vi "Actor Core.vi"(8 "Error in":errorcluster, 11 "Nested in":refnum<class "Protocol Verification Test.lvclass">) -> (0 "error out":errorcluster, 3 "Actor out":refnum<class "Actor.lvclass">)   [LabVIEW 2017, in "Protocol Verification Test.lvlib" / "Protocol Verification Test.lvclass"]
doc: "(<B>Filename</B>: Actor Framework.lvlib:Actor.lvclass:Actor Core.vi)\n\nReceives messages to the actor, reacts to them, and initiates any error handling that may shut the actor down.\n\nDescendant classes may override this VI to append parallel tasks for the actor to complete while it handles messages. Overrides use the Call Parent Method node."
uses:
  Protocol Verification Test.lvclass
  C:/Program Files (x86)/National Instruments/LabVIEW 2017/vi.lib/ActorFramework/Actor/Actor.lvclass
  <vilib>/ActorFramework/Actor/Actor.lvclass
  Proto Test Helper Loop States.ctl
  <vilib>/ActorFramework/Message Enqueuer/Message Enqueuer.lvclass
  TLV Data.ctl
  Protocol Verification Configuration.ctl
  Protocol Verification Test.lvclass/Protocol Verification Test.ctl
  <vilib>/ActorFramework/Actor/Actor.lvclass/Actor.ctl
  <vilib>/ActorFramework/Message Enqueuer/Message Enqueuer.lvclass/Message Enqueuer.ctl
  Test/Test Messages/Update Test Progress Msg/Update Test Progress Msg.lvclass/Update Test Progress Msg.ctl
  Protocol Verification Test Messages/TLV Frame Msg/TLV Frame Msg.lvclass/TLV Frame Msg.ctl
  Protocol Verification Test Messages/Write Proto Test Configuration Msg/Write Proto Test Configuration Msg.lvclass/Write Proto Test Configuration Msg.ctl
  <vilib>/ActorFramework/Message Enqueuer/Init from Existing Queue.vi
  <vilib>/ActorFramework/Message Enqueuer/Enqueue.vi
  Test/Test Messages/Update Test Progress Msg/Update Test Progress Msg.lvclass
  C:/Program Files (x86)/National Instruments/LabVIEW 2017/vi.lib/ActorFramework/Message/Message.lvclass
  Protocol Verification Test Messages/TLV Frame Msg/TLV Frame Msg.lvclass
  Protocol Verification Test Messages/Write Proto Test Configuration Msg/Write Proto Test Configuration Msg.lvclass
  <vilib>/ActorFramework/Message Priority Queue/Priority Enqueue.vi
  Test/Test/Test.lvclass
  Protocol Verification Test.lvlib
panel:
  out "Protocol Test":i32[](listbox)
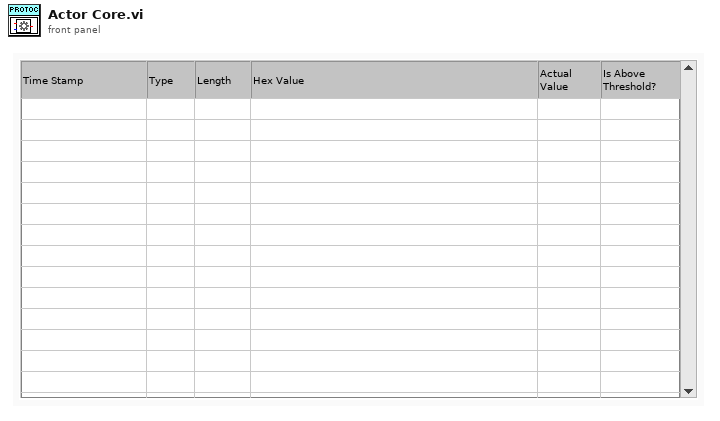
[diagram p1: front panel]
types:
  T1 = typedef "Protocol Verification Test.lvlib/TLV Data.ctl" = cluster{"Type":u8, "Length":u8, "Value":u8[]}
  T2 = typedef "Protocol Verification Test.lvlib/Protocol Verification Configuration.ctl" = cluster{"Type To Filter":i32, "Threshold":dbl, "Binary File Path":path}
  T3 = cluster{"raw bytes":u8[], "Self Enqueuer":refnum<class "Message Enqueuer.lvclass">, "TLV Data":T1[], "Test Name":string, "Protocol Verification Data":T2}
  T4 = typedef "Protocol Verification Test.lvlib/Protocol Verification Test.lvclass/Proto Test Helper Loop States.ctl" = enum16{"Poll", "Init", "Read Test Case", "Update Test Case to Actor", "Read Input File", "Parse Data", "Stream Data to Actor", "Mark End Of Stream", "Update Result", "Update Report", "Error", "Exit"}
  T5 = cluster{"Type To Filter":i32, "Threshold":dbl, "Binary File Path":string}
  T6 = typedef "Paths.ctl" = cluster{"Data Directory":path, "Test Config Dir":path, "Error Logs":path, "Event Logs":path, "Settings.Json":path, "Reports Directory":path}
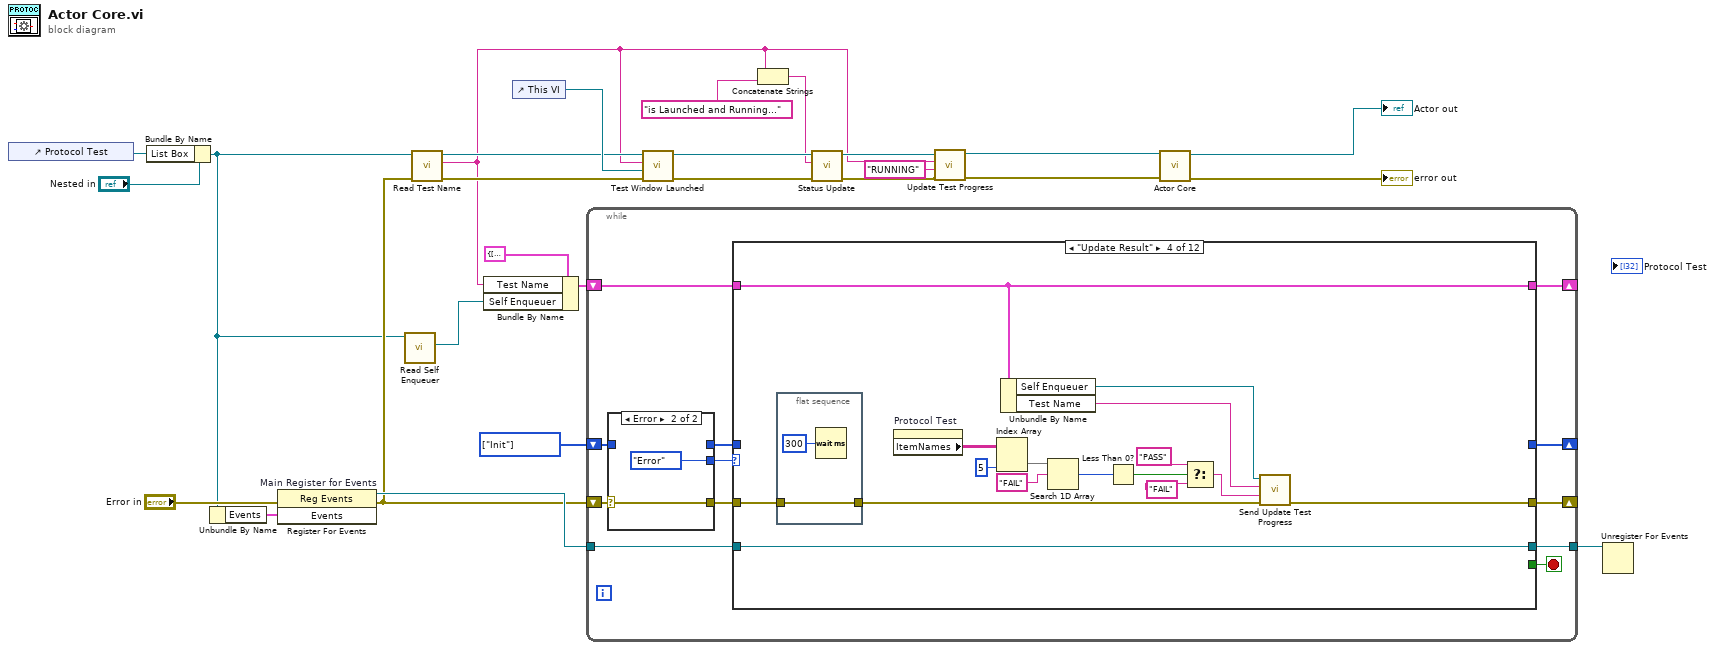
[diagram p0: block diagram]
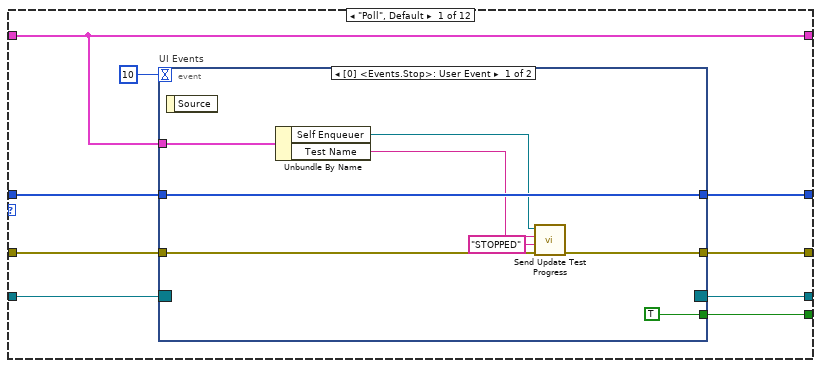
[diagram p2: hidden frame]
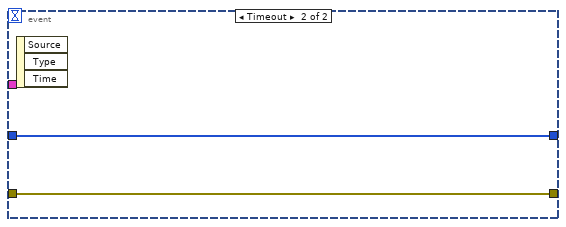
[diagram p3: hidden frame]
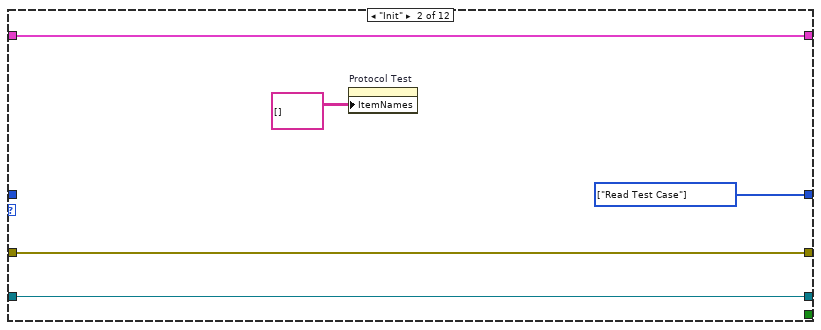
[diagram p4: hidden frame]
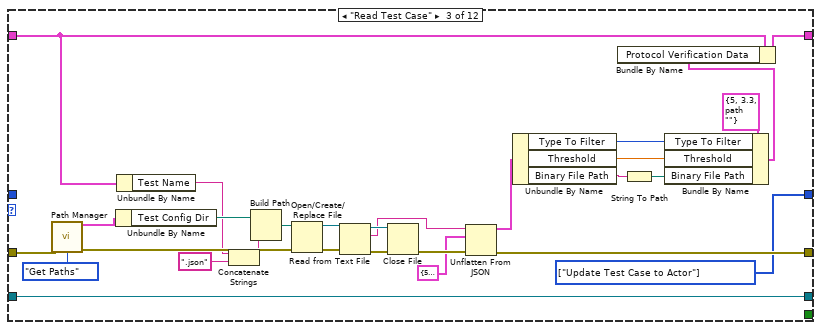
[diagram p5: hidden frame]
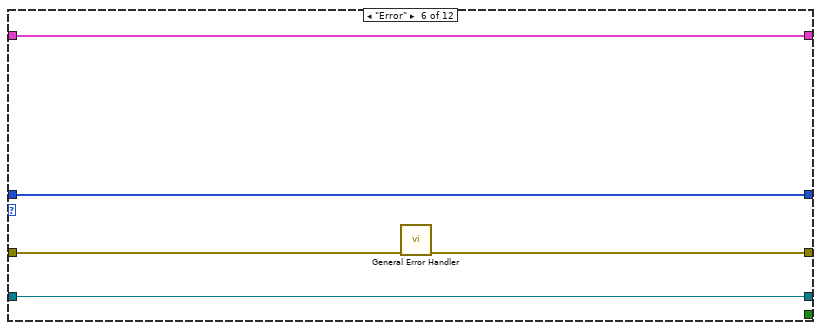
[diagram p7: hidden frame]
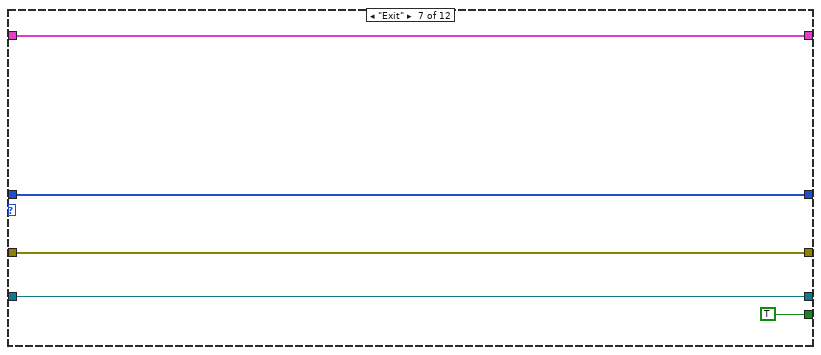
[diagram p8: hidden frame]
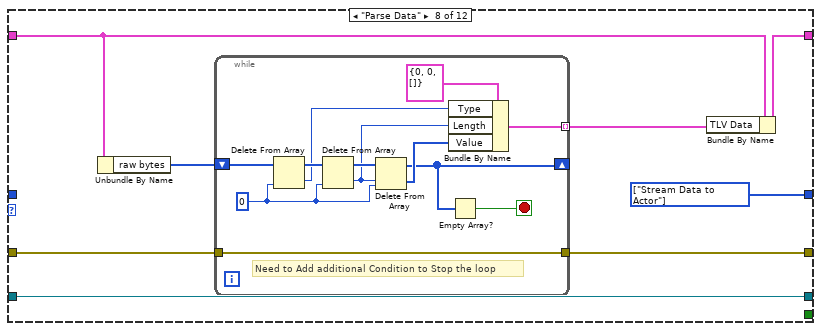
[diagram p9: hidden frame]
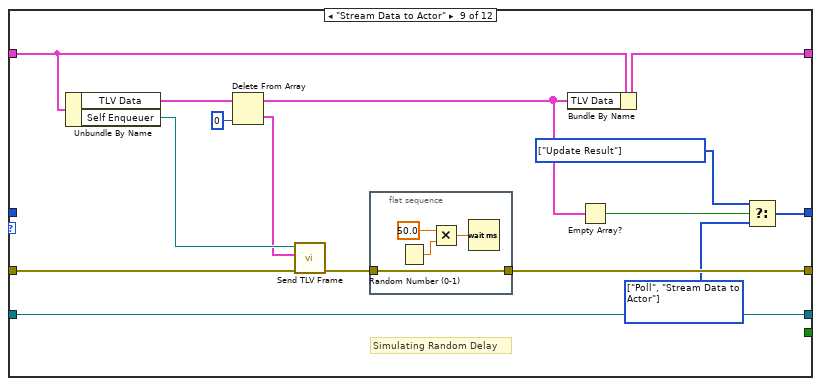
[diagram p10: hidden frame]
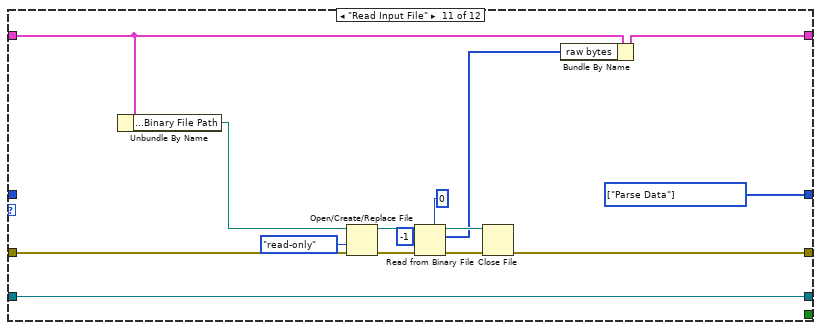
[diagram p12: hidden frame]
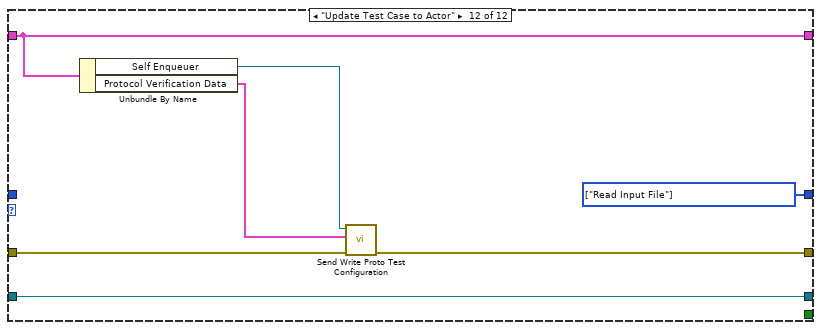
[diagram p13: hidden frame]
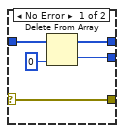
[diagram p14: hidden frame]
diagram:
  w19 = T4[] [enum."Init"] items=["Poll", "Init", "Read Test Case", "Update Test Case to Actor", "Read Input File", "Parse Data", "Stream Data to Actor", "Mark End Of Stream", "Update Result", "Update Report", "Error", "Exit"]
  n1 = control-ref of="Protocol Test"() -> (w18:refnum<vi>)
  n2 = Bundle By Name(cluster="Nested in", "List Box"=w18) -> (w5:refnum<class "Protocol Verification Test.lvclass">)
  n3 = Unbundle By Name(w5) -> ("Events"=w24:cluster{"Stop":refnum<user-event>})
  n4 = register-events "Main Register for Events"(error in="Error in", w24) -> (reference out=w25:refnum<event-registration>, error out=w7:errorcluster)  [unwired: 1 in]
  n5 = call <vilib>:"Read Self Enqueuer.vi"("Actor"=w5) -> ("Self Enqueuer"=w11:refnum<class "Message Enqueuer.lvclass">)  [unwired: 10 in]
  n6 = call-dynamic "Read Test Name.vi"("error in (no error)"=w7, "Test in"=w5) -> ("error out"=w6:errorcluster, "Test Name"=w1:string, "Test out"=w4:refnum<class "Protocol Verification Test.lvclass">)  [unwired: 7 in]
  n7 = Bundle By Name(cluster=T3 {"raw bytes"=[], "Self Enqueuer"=refnum, "TLV Data"=[], "Test Name"="", "Protocol Verification Data"={"Type To Filter"=5, "Threshold"=3.3, "Binary File Path"=path ""}}, "Test Name"=w1, "Self Enqueuer"=w11) -> (w12:T3)
  n8 = control-ref of="This VI"() -> (w21:refnum<vi>)
  n9 = while {
    tunnel: w25 -> [w39]
    tunnel: [w37] -> w23
    shift-right: [w33] -> _
    shift-left: w7 -> [w36]
    shift-right: [w32] -> _
    shift-left: w19 -> [w34]
    shift-right: [w30] -> _
    shift-left: w12 -> [w31]
    stop <- w38 stop-if-true
    n10 = case shown="Error" w36 {
      selector: w36 -> [w191 w193]
      tunnel: [w191 w193] -> w35
      tunnel: w34 -> [w190 _]
      tunnel: [w189 _] -> w28
      tunnel: [w188 Proto_Test_Helper_Loop_States."Error"] -> w29
      frame No Error {
        n11 = Delete From Array(array=w190, index=0) -> (deleted portion=w188:T4, array with subset deleted=w189:T4[])  [unwired: 1 in]
      }
      frame Error {
      }
    }
    n12 = case shown="\"Update Result\"" w29 {
      tunnel: w39 -> [w48 w63 w91 w107 w112 w117 w121 w130 w157 w164 w179 w186]
      tunnel: [w47 _ _ _ _ _ TRUE _ _ _ _ _] -> w38
      tunnel: [w46 w63 w91 w107 w112 w117 w121 w130 w157 w164 w179 w186] -> w37
      tunnel: w35 -> [w45 w62 w74 w93 _ w114 w120 w128 w150 _ w171 w185]
      tunnel: [w43 w62 w75 w106 _ w113 w120 w126 w147 _ w172 w181] -> w33
      tunnel: [w41 w60 w64 _ w110 w115 w118 w123 w144 w163 w168 w180] -> w32
      tunnel: w31 -> [w40 w59 w77 w105 w111 w116 w119 w129 w156 w162 w167 w184]
      tunnel: [w40 w59 w66 w105 w111 w116 w119 w125 w155 w162 w170 w184] -> w30
      tunnel: w28 -> [w42 _ _ _ w110 w115 w118 _ _ w163 _ _]
      frame "Poll", Default {
        n13 = event "UI Events" shown="[0] <Events.Stop>: User Event" {
          selector: w48 -> [_ _]
          dyn-events: [_ _] -> w46
          timeout: 10 -> [_ _]
          tunnel: [TRUE _] -> w47
          tunnel: w45 -> [w52 w58]
          tunnel: [w51 w58] -> w43
          tunnel: w42 -> [w55 w57]
          tunnel: [w55 w57] -> w41
          tunnel: w40 -> [w50 _]
          event User Event {
            n14 = event-data() -> ()  [unwired: 1 in, 1 out]
            n15 = Unbundle By Name(w50) -> ("Self Enqueuer"=w54:refnum<class "Message Enqueuer.lvclass">, "Test Name"=w53:string)
            n16 = call "Send Update Test Progress.vi"("error in (no error)"=w52, "State"="STOPPED", "Test Name"=w53, "Message Enqueuer"=w54) -> ("error out"=w51:errorcluster)  [unwired: 6 in, 1 out]
          }
          event Timeout {
            n17 = event-data() -> ()  [unwired: 1 in, 3 out]
          }
        }
      }
      frame "Init" {
        w60 = T4[] [enum."Read Test Case"] items=["Poll", "Init", "Read Test Case", "Update Test Case to Actor", "Read Input File", "Parse Data", "Stream Data to Actor", "Mark End Of Stream", "Update Result", "Update Report", "Error", "Exit"]
        n18 = property on="Protocol Test" class="MCListbox (strict)"("ItemNames"=string[][] [] ("Item Names")) -> ()  [unwired: 2 in, 2 out]
      }
      frame "Read Test Case" {
        w64 = T4[] [enum."Update Test Case to Actor"] items=["Poll", "Init", "Read Test Case", "Update Test Case to Actor", "Read Input File", "Parse Data", "Stream Data to Actor", "Mark End Of Stream", "Update Result", "Update Report", "Error", "Exit"] ("f")
        n19 = call "Path Manager.vi"("Error in (no error)"=w74, "Options"=enum16{"Get Paths", "Init Paths"}."Get Paths") -> ("Cluster"=w82:T6, "Error out"=w84:errorcluster)  [unwired: 12 in]
        n20 = Unbundle By Name(w82) -> ("Test Config Dir"=w81:path)
        n21 = Unbundle By Name(w77) -> ("Test Name"=w76:string)
        n22 = Concatenate Strings(w76, ".json" ("string")) -> (w80:string)
        n23 = Build Path(base path=w81, name or relative path=w80) -> (appended path=w78:path)
        n24 = Open/Create/Replace File(file path (use dialog)=w78, error in=w84) -> (refnum out=w90:refnum<file>, error out=w87:errorcluster)  [unwired: 4 in, 1 out]
        n25 = Read from Text File(file (use dialog)=w90, error in=w87) -> (refnum out=w88:refnum<file>, text=w85:string, error out=w89:errorcluster)  [unwired: 2 in, 1 out]
        n26 = Close File(refnum=w88, error in=w89) -> (error out=w86:errorcluster)  [unwired: 1 out]
        n27 = Unflatten From JSON(JSON string=w85, type and defaults=T5 {"Type To Filter"=5, "Threshold"=3.3, "Binary File Path"=""} ("Cluster"), error in (no error)=w86) -> (value=w71:T5, error out=w75:errorcluster)  [unwired: 4 in]
        n28 = Unbundle By Name(w71) -> ("Type To Filter"=w70:i32, "Threshold"=w69:dbl, "Binary File Path"=w68:string)
        n29 = String To Path(string=w68) -> (path=w67:path)
        n30 = Bundle By Name(cluster=T2 {"Type To Filter"=5, "Threshold"=3.3, "Binary File Path"=path ""} ("Cluster"), "Type To Filter"=w70, "Threshold"=w69, "Binary File Path"=w67) -> (w65:T2)
        n31 = Bundle By Name(cluster=w77, "Protocol Verification Data"=w65) -> (w66:T3)
      }
      frame "Update Result" {
        n32 = flat-sequence {
          tunnel: w93 -> [w109]
          tunnel: [w109] -> w92
          frame #0 {
            n33 = Wait (ms)(milliseconds to wait=u32 300) -> ()  [unwired: 1 out]
          }
        }
        n34 = property on="Protocol Test" class="MCListbox (strict)"() -> ("ItemNames"=w102:string[][])  [unwired: 2 in, 2 out]
        n35 = Index Array(array=w102, index (col)=5 ("disabled index (col)")) -> (element=w100:string[])  [unwired: 1 in]
        n36 = Unbundle By Name(w105) -> ("Self Enqueuer"=w104:refnum<class "Message Enqueuer.lvclass">, "Test Name"=w103:string)
        n37 = Search 1D Array(1D array=w100, element="FAIL") -> (index of element=w98:i32)  [unwired: 1 in]
        n38 = Less Than 0?(x=w98) -> (x < 0?=w97:bool)
        n39 = Select(t="PASS" ("State"), s=w97, f="FAIL" ("State")) -> (s? t:f=w94:string)
        n40 = call "Send Update Test Progress.vi"("error in (no error)"=w92, "State"=w94, "Test Name"=w103, "Message Enqueuer"=w104) -> ("error out"=w106:errorcluster)  [unwired: 6 in, 1 out]
      }
      frame "Update Report" {
      }
      frame "Error" {
        n41 = call <vilib>:"General Error Handler.vi"("error in (no error)"=w114) -> ("error out"=w113:errorcluster)  [unwired: 10 in, 4 out]
      }
      frame "Exit" {
      }
      frame "Parse Data" {
        w123 = T4[] [enum."Stream Data to Actor"] items=["Poll", "Init", "Read Test Case", "Update Test Case to Actor", "Read Input File", "Parse Data", "Stream Data to Actor", "Mark End Of Stream", "Update Result", "Update Report", "Error", "Exit"] ("f")
        n42 = Unbundle By Name(w129) -> ("raw bytes"=w127:u8[])
        n43 = while {
          tunnel: w128 -> [w134]
          shift-right: [w131] -> _
          shift-left: w127 -> [w141]
          tunnel: [w134] -> w126
          tunnel: [w133] -> w124 mode=indexing
          stop <- w138 stop-if-true
          w142 = 0 ("index")
          # "Need to Add additional Condition to Stop the loop"
          n44 = Delete From Array(array=w141, index=w142) -> (deleted portion=w136:u8, array with subset deleted=w140:u8[])  [unwired: 1 in]
          n45 = Delete From Array(array=w140, index=w142) -> (deleted portion=w135:u8, array with subset deleted=w139:u8[])  [unwired: 1 in]
          n46 = Delete From Array(array=w139, length=w135, index=w142) -> (deleted portion=w132:u8[], array with subset deleted=w131:u8[])
          n47 = Bundle By Name(cluster=T1 {"Type"=0, "Length"=0, "Value"=[]} ("Cluster"), "Type"=w136, "Length"=w135, "Value"=w132) -> (w133:T1)
          n48 = Empty Array?(array=w131) -> (empty?=w138:bool)
        }
        n49 = Bundle By Name(cluster=w129, "TLV Data"=w124) -> (w125:T3)
      }
      frame "Stream Data to Actor" {
        w143 = T4[] [enum."Poll", enum."Stream Data to Actor"] items=["Poll", "Init", "Read Test Case", "Update Test Case to Actor", "Read Input File", "Parse Data", "Stream Data to Actor", "Mark End Of Stream", "Update Result", "Update Report", "Error", "Exit"] ("f")
        w145 = T4[] [enum."Update Result"] items=["Poll", "Init", "Read Test Case", "Update Test Case to Actor", "Read Input File", "Parse Data", "Stream Data to Actor", "Mark End Of Stream", "Update Result", "Update Report", "Error", "Exit"] ("t")
        # "Simulating Random Delay"
        n50 = Unbundle By Name(w156) -> ("TLV Data"=w154:T1[], "Self Enqueuer"=w152:refnum<class "Message Enqueuer.lvclass">)
        n51 = Delete From Array(array=w154, index=0 ("length")) -> (deleted portion=w151:T1, array with subset deleted=w149:T1[])  [unwired: 1 in]
        n52 = call "Send TLV Frame.vi"("error in (no error)"=w150, "TLV Frame"=w151, "Message Enqueuer"=w152) -> ("error out"=w148:errorcluster)  [unwired: 7 in, 1 out]
        n53 = flat-sequence {
          tunnel: w148 -> [w161]
          tunnel: [w161] -> w147
          frame #0 {
            n54 = Random Number (0-1)() -> (number: 0 to 1=w160:dbl)
            n55 = Multiply(x=50.0, y=w160) -> (x*y=w158:dbl)
            n56 = Wait (ms)(milliseconds to wait=w158) -> ()  [unwired: 1 out]
          }
        }
        n57 = Bundle By Name(cluster=w156, "TLV Data"=w149) -> (w155:T3)
        n58 = Empty Array?(array=w149) -> (empty?=w146:bool)
        n59 = Select(t=w145, s=w146, f=w143) -> (s? t:f=w144:T4[])
      }
      frame "Mark End Of Stream" {
      }
      frame "Read Input File" {
        w168 = T4[] [enum."Parse Data"] items=["Poll", "Init", "Read Test Case", "Update Test Case to Actor", "Read Input File", "Parse Data", "Stream Data to Actor", "Mark End Of Stream", "Update Result", "Update Report", "Error", "Exit"]
        n60 = Unbundle By Name(w167) -> ("Protocol Verification Data.Binary File Path"=w166:path)
        n61 = Open/Create/Replace File(file path (use dialog)=w166, error in=w171, access (0:read/write)=enum16{"read/write", "read-only", "write-only"}."read-only") -> (refnum out=w178:refnum<file>, error out=w177:errorcluster)  [unwired: 3 in, 1 out]
        n62 = Read from Binary File(5:u8 0, 8:w177, 10:-1 ("count (1)"), 11:w178) -> (0:w173:errorcluster, 2:w169:u8[], 3:w174:refnum<file>)  [unwired: 2 in, 1 out]
        n63 = Close File(refnum=w174, error in=w173) -> (error out=w172:errorcluster)  [unwired: 1 out]
        n64 = Bundle By Name(cluster=w167, "raw bytes"=w169) -> (w170:T3)
      }
      frame "Update Test Case to Actor" {
        w180 = T4[] [enum."Read Input File"] items=["Poll", "Init", "Read Test Case", "Update Test Case to Actor", "Read Input File", "Parse Data", "Stream Data to Actor", "Mark End Of Stream", "Update Result", "Update Report", "Error", "Exit"] ("f")
        n65 = Unbundle By Name(w184) -> ("Self Enqueuer"=w183:refnum<class "Message Enqueuer.lvclass">, "Protocol Verification Data"=w182:T2)
        n66 = call "Send Write Proto Test Configuration.vi"("error in (no error)"=w185, "Cluster"=w182, "Message Enqueuer"=w183) -> ("error out"=w181:errorcluster)  [unwired: 7 in, 1 out]
      }
    }
  }
  n67 = call-dynamic "Test Window Launched.vi"("error in (no error)"=w6, "VI Refnum"=w21, "Window Name"=w1, "Test in"=w4) -> ("error out"=w16:errorcluster, "Test out"=w17:refnum<class "Protocol Verification Test.lvclass">)  [unwired: 6 in]
  n68 = Concatenate Strings(w1, "is Launched and Running..." ("string")) -> (w14:string)
  n69 = call-dynamic "Status Update.vi"("error in (no error)"=w16, "Status"=w14, "Test in"=w17) -> ("error out"=w9:errorcluster, "Test out"=w10:refnum<class "Protocol Verification Test.lvclass">)  [unwired: 7 in]
  n70 = call-dynamic "Update Test Progress.vi"("error in (no error)"=w9, "State"="RUNNING", "Test Name"=w1, "Test in"=w10) -> ("error out"=w3:errorcluster, "Test out"=w2:refnum<class "Protocol Verification Test.lvclass">)  [unwired: 6 in]
  n71 = call-parent "Actor Core.vi"("error in"=w3, "Actor in"=w2) -> ("error out"=→"error out":errorcluster, "Actor out"=→"Actor out":refnum<class "Actor.lvclass">)  [unwired: 8 in]
  n72 = Unregister For Events(event registration refnum=w23) -> ()  [unwired: 1 in, 1 out]
